vi "_022.vi"() -> ()   [LabVIEW 2024]
panel:
  in  "Array":T1(array[cluster])
  # "How to put cluster in to Array ?"
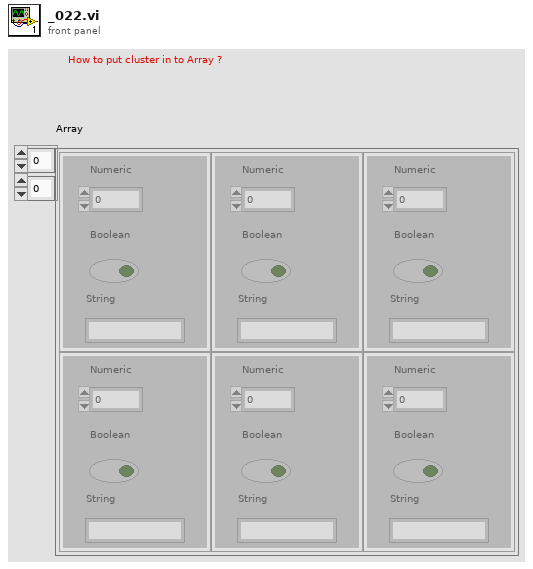
[diagram p1: front panel]
types:
  T1 = cluster{"Numeric":dbl, "Boolean":bool, "String":string}[][]
  T2 = cluster{"Numeric":dbl, "Boolean":bool, "String":string}[]
  T3 = cluster{"Array[0]":cluster{"Numeric":dbl, "Boolean":bool, "String":string}, "Array[1]":cluster{"Numeric":dbl, "Boolean":bool, "String":string}, "Array[2]":cluster{"Numeric":dbl, "Boolean":bool, "String":string}, "Array[3]":cluster{"Numeric":dbl, "Boolean":bool, "String":string}, "Array[4]":cluster{"Numeric":dbl, "Boolean":bool, "String":string}, "Array[5]":cluster{"Numeric":dbl, "Boolean":bool, "String":string}, "Array[6]":cluster{"Numeric":dbl, "Boolean":bool, "String":string}, "Array[7]":cluster{"Numeric":dbl, "Boolean":bool, "String":string}, "Array[8]":cluster{"Numeric":dbl, "Boolean":bool, "String":string}}
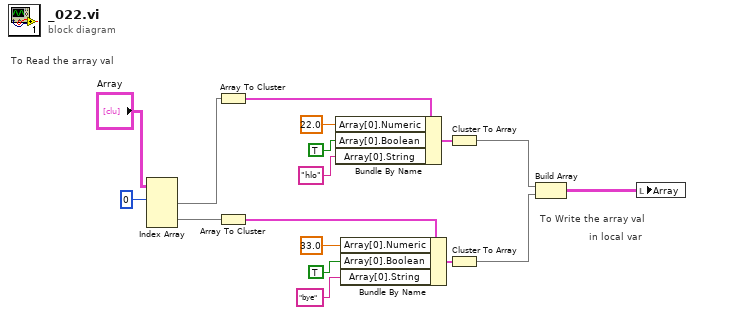
[diagram p0: block diagram]
diagram:
  # "in local var"
  # "To Write the array val"
  # "To Read the array val"
  n1 = Index Array "Index Array"(array="Array", index (row) #1=0 ("index")) -> (element #1=w15:T2, element #2=w4:T2)  [unwired: 3 in]
  n2 = Array To Cluster(array=w15) -> (cluster=w14:T3)
  n3 = Array To Cluster(array=w4) -> (cluster=w3:T3)
  n4 = Bundle By Name "Bundle By Name"(cluster=w14, "Array[0].Numeric"=22.0, "Array[0].Boolean"=TRUE, "Array[0].String"="hlo") -> (w10:T3)
  n5 = Bundle By Name "Bundle By Name"(cluster=w3, "Array[0].Numeric"=33.0, "Array[0].Boolean"=TRUE, "Array[0].String"="bye") -> (w2:T3)
  n6 = Cluster To Array(cluster=w10) -> (array=w9:T2)
  n7 = Cluster To Array(cluster=w2) -> (array=w1:T2)
  n8 = Build Array "Build Array"(w9, w1) -> (w8:T1)
  n9 = local write "Array"(w8) -> ()
